vi "PH_GetCamInformation.PC Get Info.vi"(2 "MCL Listbox GUI Ref":refnum<vi>, 5 "error in":errorcluster) -> (19 "error out":errorcluster)   [LabVIEW 2014, in "PH_GetCamInformation.lvlib"]
doc: "This is the proc case \"get information\"."
uses:
  PH_GetCamInformation.lvlib
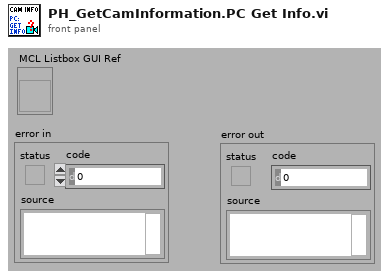
[diagram p1: front panel]
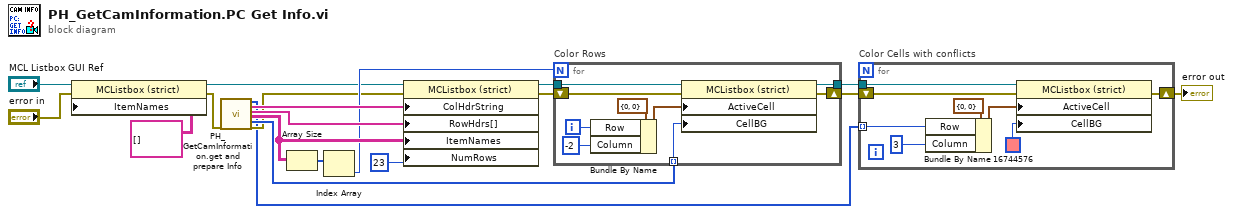
[diagram p0: block diagram]
diagram:
  n1 = property class="MCListbox (strict)"(reference="MCL Listbox GUI Ref", error in="error in", "ItemNames"=string[][] [] ("Item Names")) -> (reference out=w9:refnum<vi>, error out=w6:errorcluster)
  n2 = call "PH_GetCamInformation.get and prepare Info.vi"("error in"=w6) -> ("Rows with conflicts"=w2:i32[], "ColHdrs[]"=w17:string[], "RowHdrs[]"=w16:string[], "ItemNames"=w18:string[][], "Row Cell BG"=w19:u32[], "error out"=w5:errorcluster)  [unwired: 13 in]
  n3 = Array Size(array=w18) -> (size(s)=w15:i32[])
  n4 = Index Array(array=w15) -> (element=w11:i32)  [unwired: 1 in]
  n5 = property class="MCListbox (strict)"(reference=w9, error in=w5, "ColHdrString"=w17, "RowHdrs[]"=w16, "ItemNames"=w18, "NumRows"=u32 23 ("Number of Rows")) -> (reference out=w12:refnum<vi>, error out=w13:errorcluster)
  n6 = for "Color Rows" {
    N: w11 -> [_]
    tunnel: w12 -> [w26]
    shift-right: [w27] -> w4
    shift-left: w13 -> [w28]
    tunnel: w19 -> [w23] mode=indexing
    tunnel: [w20] -> w1
    i -> [w22]
    n7 = Bundle By Name(cluster=cluster{"Row":i32, "Column":i32} {"Row"=0, "Column"=0} ("Active Cell:Active Cell"), "Row"=w22, "Column"=-2 ("Row")) -> (w25:cluster{"Row":i32, "Column":i32})
    n8 = property class="MCListbox (strict)"(reference=w26, error in=w28, "ActiveCell"=w25, "CellBG"=w23) -> (reference out=w20:refnum<vi>, error out=w27:errorcluster)
  }
  n9 = for "Color Cells with conflicts" {
    tunnel: w1 -> [w34]
    tunnel: w2 -> [w33] mode=indexing
    shift-right: [w35] -> w3
    shift-left: w4 -> [w36]
    n10 = Bundle By Name(cluster=cluster{"Row":i32, "Column":i32} {"Row"=0, "Column"=0} ("Active Cell:Active Cell"), "Row"=w33, "Column"=3 ("Row")) -> (w32:cluster{"Row":i32, "Column":i32})
    n11 = property class="MCListbox (strict)"(reference=w34, error in=w36, "ActiveCell"=w32, "CellBG"=u32 16744576 ("Color Box")) -> (error out=w35:errorcluster)  [unwired: 1 out]
  }
  "error out" <- w3
